vi "Main.vi"() -> ()   [LabVIEW 2020]
uses:
  TypeDefs/Enum_MainQueueElements.ctl
  TypeDefs/Refs_Common.ctl
  <vilib>/Stadlmann TEC/OXYGEN Datastream/VIs/Data Aquasation/TypeDefs/DataPoint_Double.ctl
  <vilib>/event_ctls.llb/eventvkey.ctl
  TypeDefs/TD_Case_SimpleFGVModes.ctl
  TypeDefs/Enum_CmdPromptActions.ctl
  <vilib>/Stadlmann TEC/OXYGEN Datastream/VIs/Setup/TypeDefs/States.ctl
  <vilib>/Stadlmann TEC/OXYGEN Datastream/VIs/Channel List Access/SubVIs/ChannelList_GetNames.vi
  <vilib>/Stadlmann TEC/OXYGEN Datastream/VIs/Setup/SubVIs/Start_Group.vi
  <vilib>/Stadlmann TEC/OXYGEN Datastream/VIs/Setup/SubVIs/Stop_Group.vi
  <vilib>/Stadlmann TEC/OXYGEN Datastream/VIs/Setup/SubVIs/Port_set.vi
  <vilib>/Stadlmann TEC/OXYGEN Datastream/VIs/Setup/SubVIs/Port_get.vi
  <vilib>/Stadlmann TEC/OXYGEN Datastream/VIs/Setup/SubVIs/Items_set.vi
  <vilib>/Stadlmann TEC/OXYGEN Datastream/VIs/Setup/SubVIs/Init_Group.vi
  <vilib>/Stadlmann TEC/OXYGEN Datastream/OXYGEN_Datastream.lvlib
  VIs/VI_ReadData.vi
panel:
  out "Bool_StatusLED":bool=TRUE
  in  "STR_HostAddress":string="127.0.0.1:10001"
  in  "Button_Disconnect":bool
  in  "Button_Connect":bool
  in  "Button_querryChs":bool
  in  "LBox_ChList":i32(listbox)
  in  "Datastream Port":u32=10003
  in  "Button_Set_Port":bool
  in  "Button_Reset":bool
  in  "Button_Init":bool
  in  "Button_Get_State":bool
  in  "Button_Get_Port":bool
  in  "Button_Start":bool
  in  "Button_Stop":bool
  in  "User Commands":string
  in  "STR_ChName1":string
  out "Num_ChValue1":dbl format="%04.3g"
  in  "STR_ChName2":string
  out "Num_ChValue2":dbl format="%1.3g"
  in  "STR_ChName3":string
  out "Num_ChValue3":dbl format="%1.3g"
  in  "STR_ChName4":string
  out "Num_ChValue4":dbl format="%.3g"
  in  "STR_ChName5":string
  out "Num_ChValue5":dbl format="%.3g"
  in  "STR_ChName6":string
  out "Num_ChValue6":dbl format="%.3g"
  out "Recorder":T1(graph)
  out "STR_CmdPrompt":string
  # "IP Address/Hostname and Port Number \n                Example:  xxx.xxx.xxx.xxx:yyyyy"
  # "Datastream Group 1"
  # "Channel 1"
  # "Channel 3"
  # "Channel 2"
  # "Channel 5"
  # "Channel 4"
  # "Channel 6"
  # "Channel 1"
  # "Channel 2"
  # "Channel 3"
  # "Channel 4"
  # "Channel 5"
  # "Channel 6"
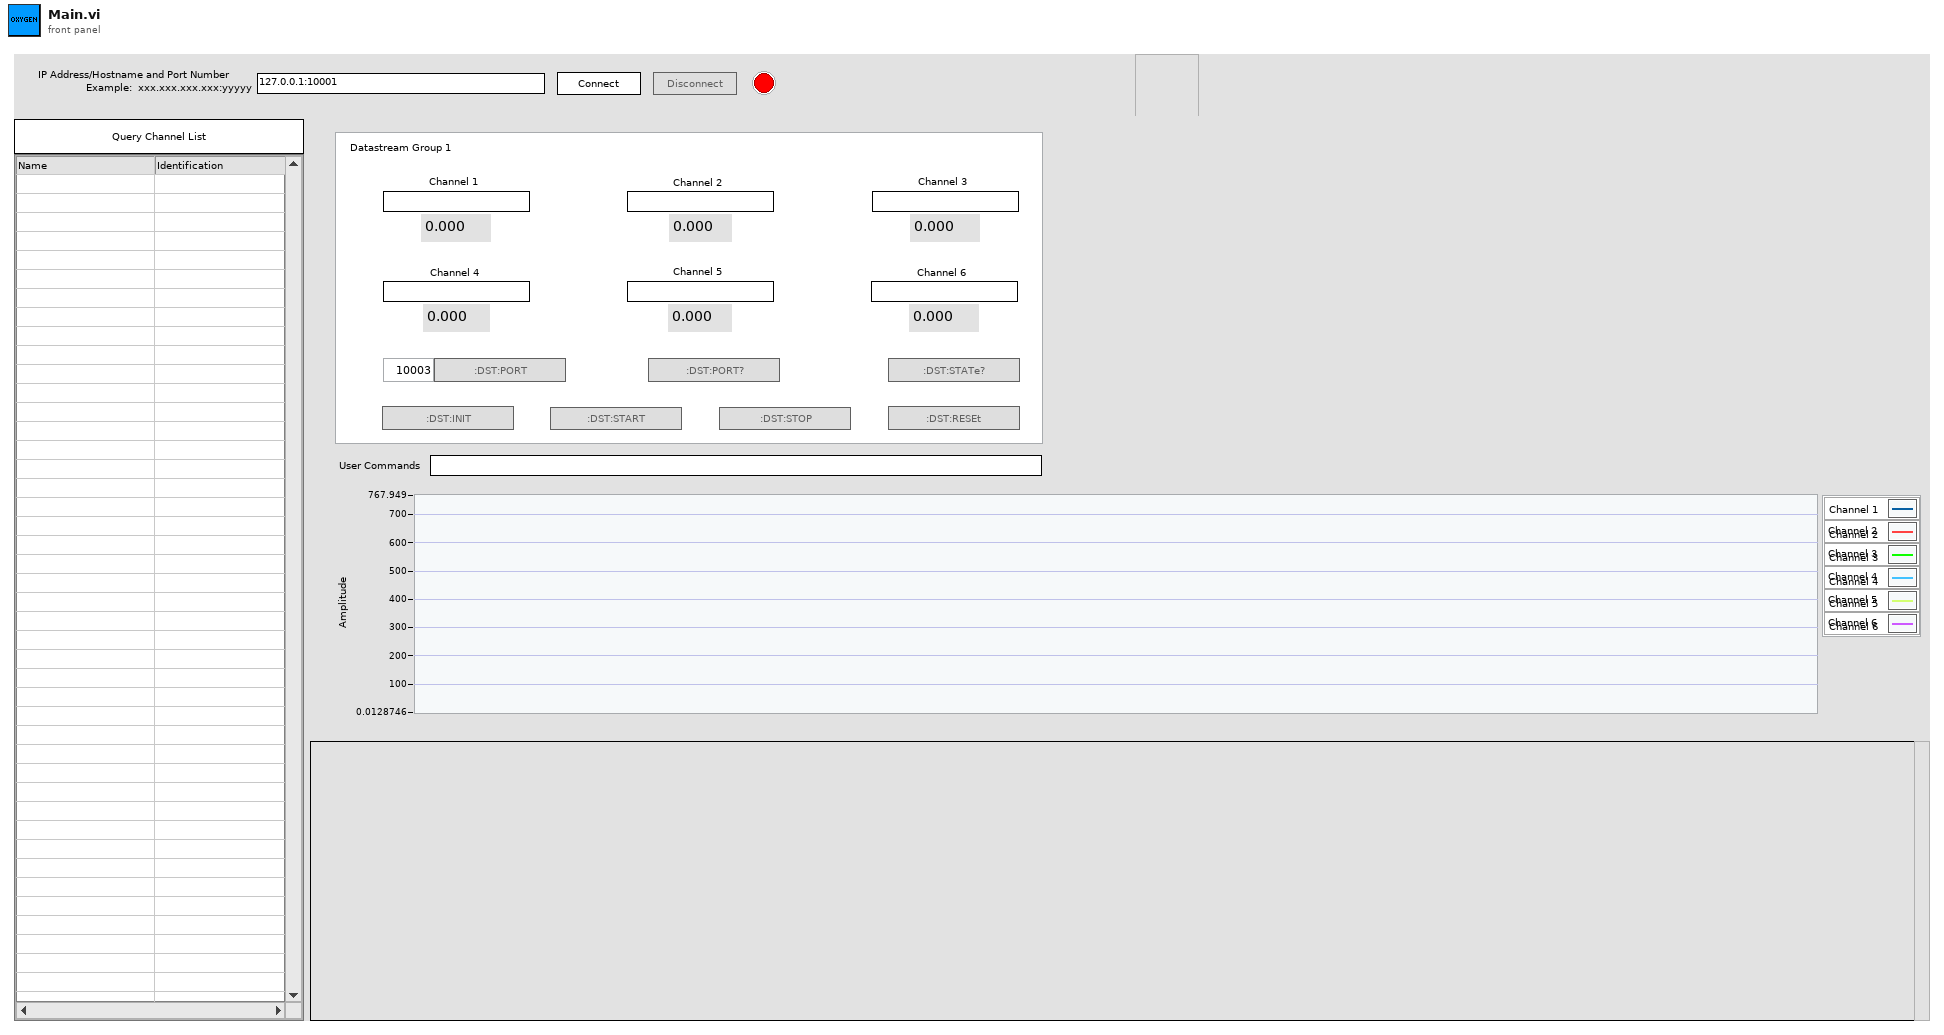
[diagram p1: front panel]
types:
  T1 = cluster{"DataPoints":cluster{"Value":dbl, "Time":dbl}[]}[]
  T2 = typedef "OXYGEN_Datastream.lvlib/DataPoint_Double.ctl" = cluster{"DataPoints":cluster{"Time":dbl, "Value":dbl}[]}
  T3 = typedef "Refs_Common.ctl" = cluster{"LBox_ChList":refnum<vi>, "OXY_SCPI Ref":refnum<visa-resource-name>, "STR_ChName1":refnum<vi>, "STR_ChName2":refnum<vi>, "STR_ChName3":refnum<vi>, "STR_ChName4":refnum<vi>, "STR_ChName5":refnum<vi>, "STR_ChName6":refnum<vi>, "Button_Stop":refnum<vi>, "Button_Start":refnum<vi>, "Button_Disconnect":refnum<vi>, "Button_Connect":refnum<vi>, "Bool_StatusLED":refnum<vi>, "DS Ref":refnum<visa-resource-name>, "Button_SetPort":refnum<vi>, "Button_GetPort":refnum<vi>, "Button_GetState":refnum<vi>, "Button_Reset":refnum<vi>, "Button_Init":refnum<vi>, "STR_UserCMD":refnum<vi>, "STR_CmdPromp":refnum<vi>, "Port":refnum<vi>, "Button_QuerryChs":refnum<vi>, "Graph":refnum<vi>, "STR_ConnAddress":refnum<vi>}
  T4 = typedef "Enum_MainQueueElements.ctl" = enum16{"Timeout", "Init", "Button_Reset_Pressed", "Button_QuerryChList_Pressed", "Button_UsrCmdSet_Pressed", "Button_StartTransfer_Pressed", "Button_StopTransfer_Pressed", "Button_Connect_Pressed", "Button_Disconnect_Pressed", "Button_SetPort_Presssed", "Button_GetPort_Pressed", "Button_GetState_Pressed", "Button_Init_Pressed", "NewDragAndDrop", "CloseApp"}
  T5 = typedef "Enum_CmdPromptActions.ctl" = enum16{"Init", "Add", "EditSettings", "Close"}
  T6 = cluster{"send_data":string, "received_data":string}
  T7 = typedef "OXYGEN_Datastream.lvlib/States.ctl" = enum16{"Invalid", "Config", "Initialized", "Running", "Error", "Unlicensed"}
  T8 = enum8{"Enabled", "Disabled", "Disabled and Grayed Out"}
  T9 = typedef "TD_Case_SimpleFGVModes.ctl" = enum16{"Set", "Get"}
  T10 = typedef "OXYGEN_Datastream.lvlib/Cluster_RawCommData.ctl" = cluster{"send_data":string, "received_data":string}
  T11 = typedef "eventvkey.ctl" = enum16{"ASCII", "Enter", "Return", "Shift", "Ctrl", "Alt", "Cmd", "Opt", "Caps", "NumLock", "Clear", "Break", "Up", "Down", "Left", "Right", "Insert", "Delete", "Home", "End", "PageUp", "PageDown", "Escape", "Help", "Pause", "ScrollLock", "F1", "F2", "F3", "F4", "F5", "F6", "F7", "F8", "F9", "F10", "F11", "F12", "F13", "F14", "F15", "F16", "F17", "F18", "F19", "F20", "F21", "F22", "F23", "F24", "Play", "VolumeUp", "VolumeDown", "Mute", "Two Byte Char"}
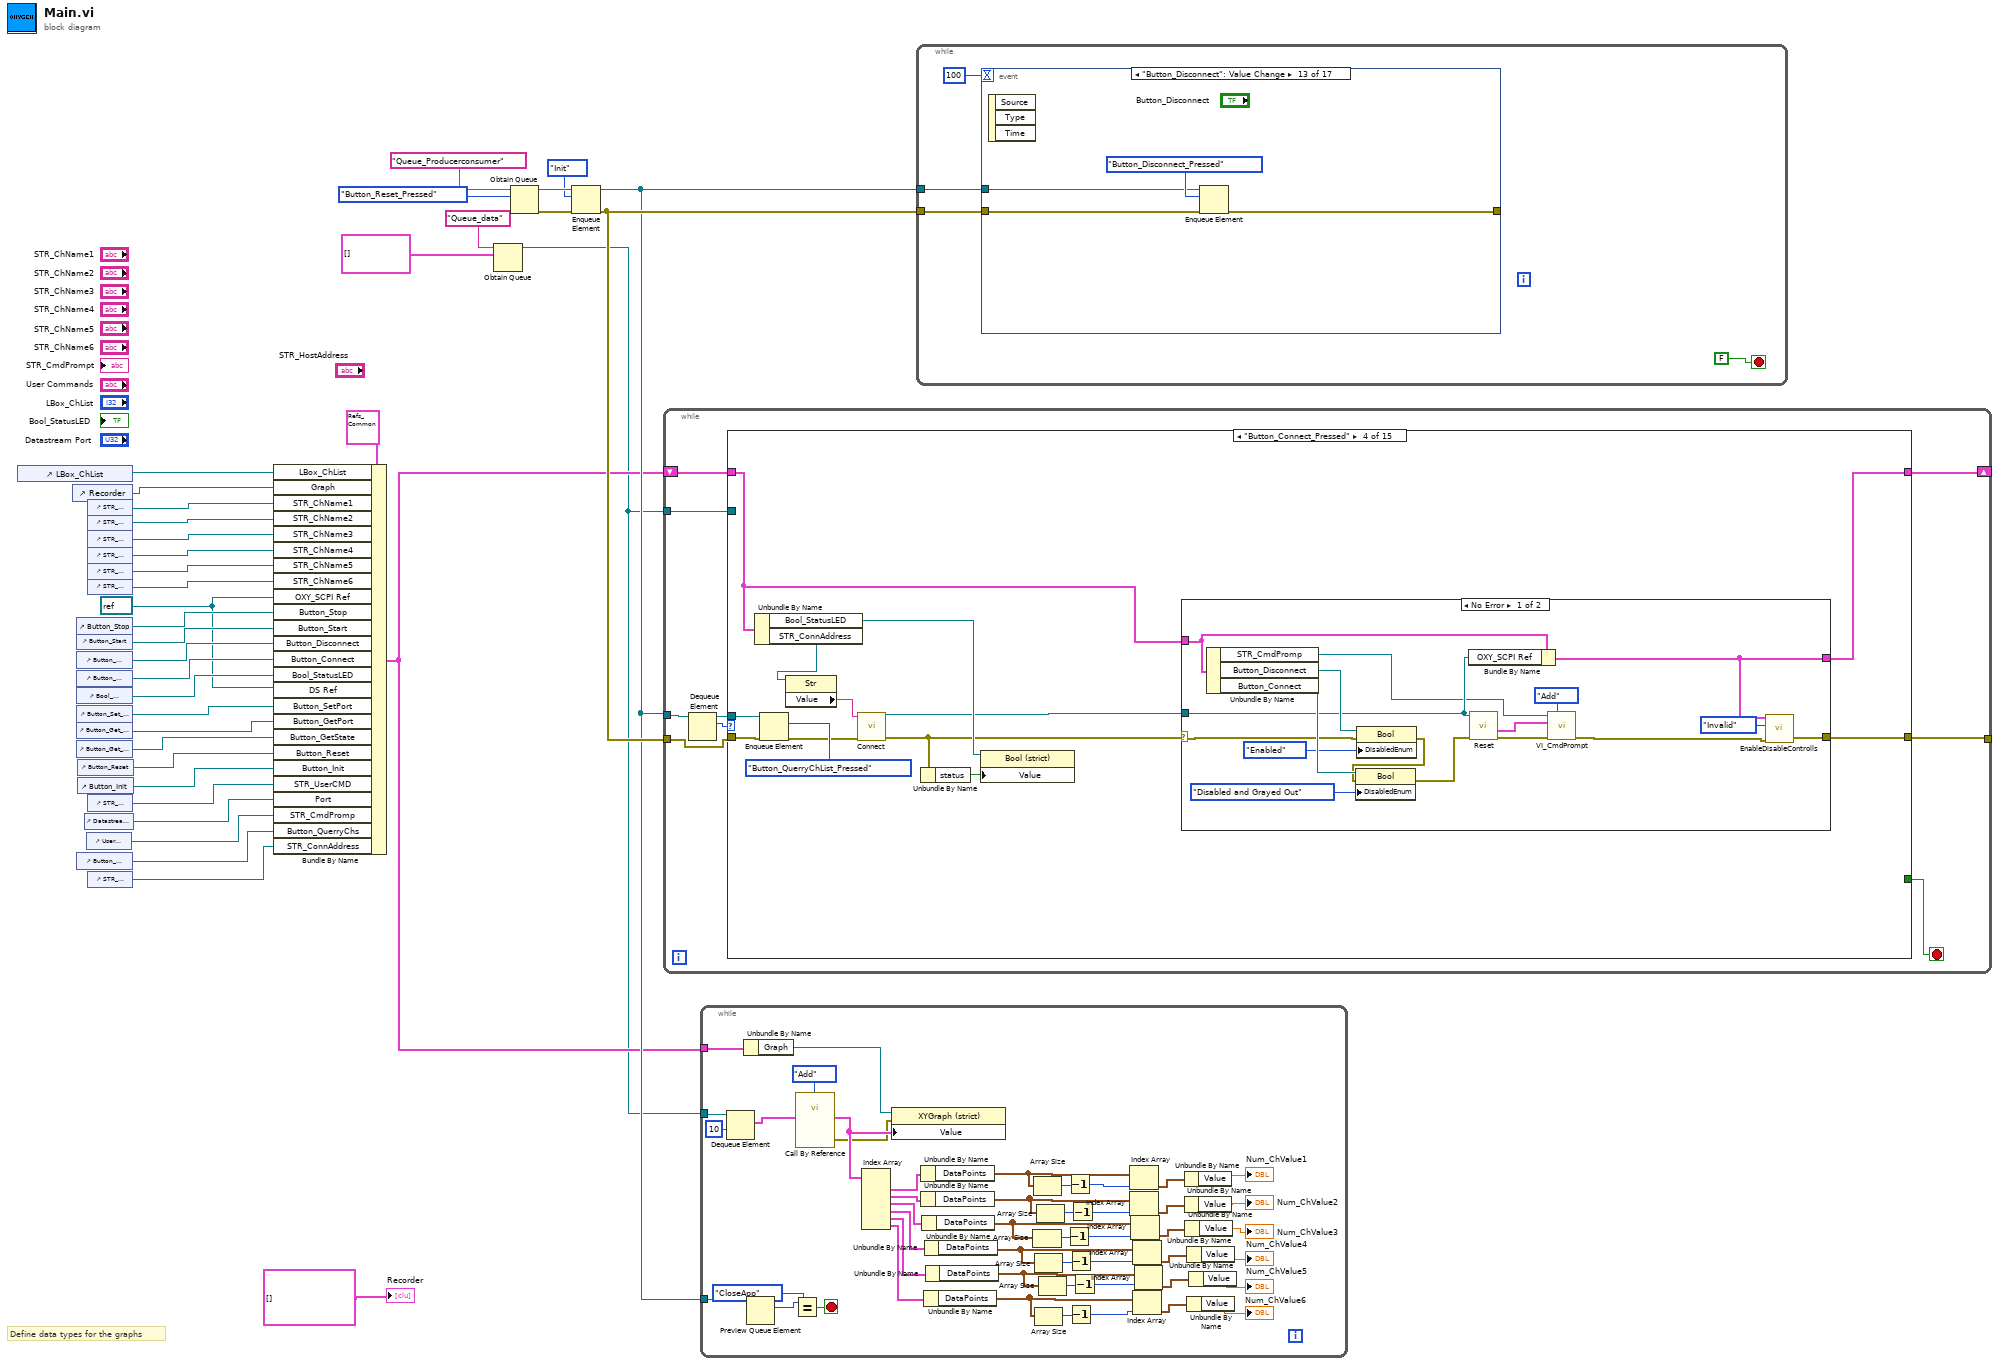
[diagram p0: block diagram]
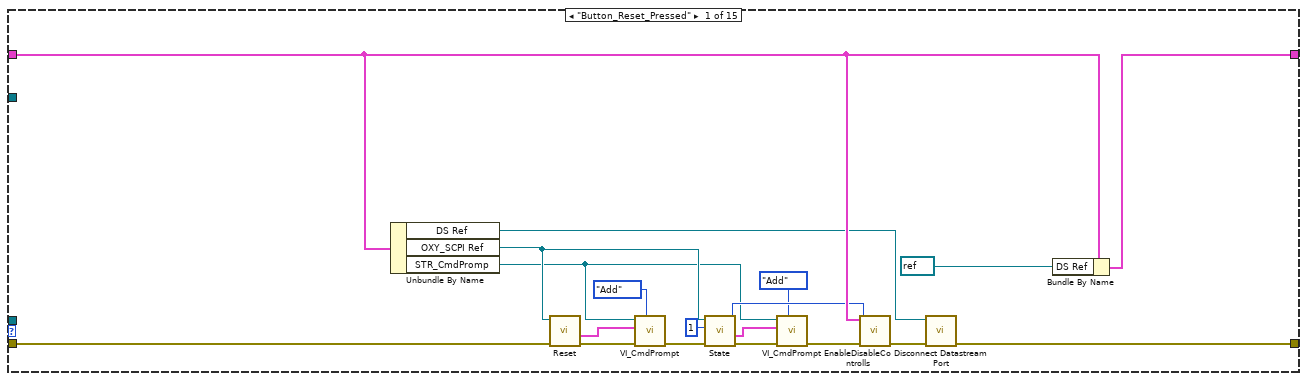
[diagram p2: hidden frame]
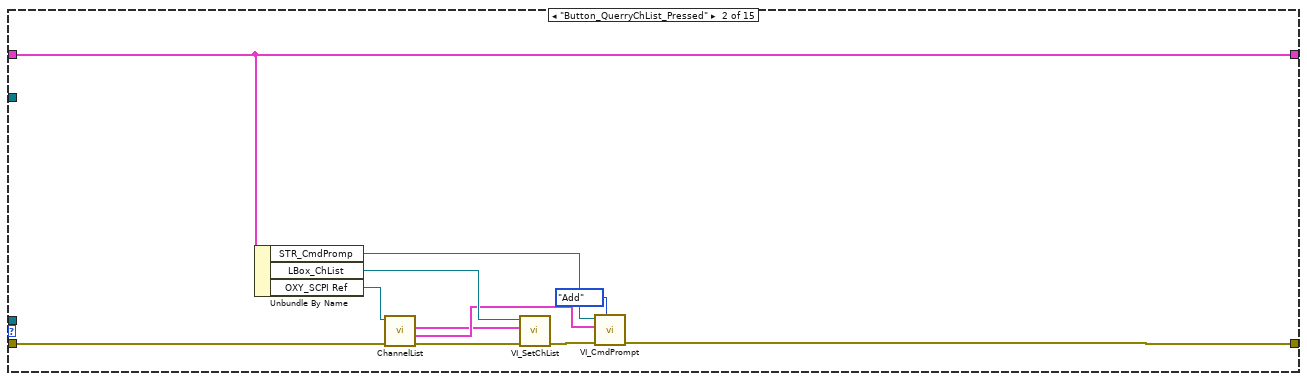
[diagram p3: hidden frame]
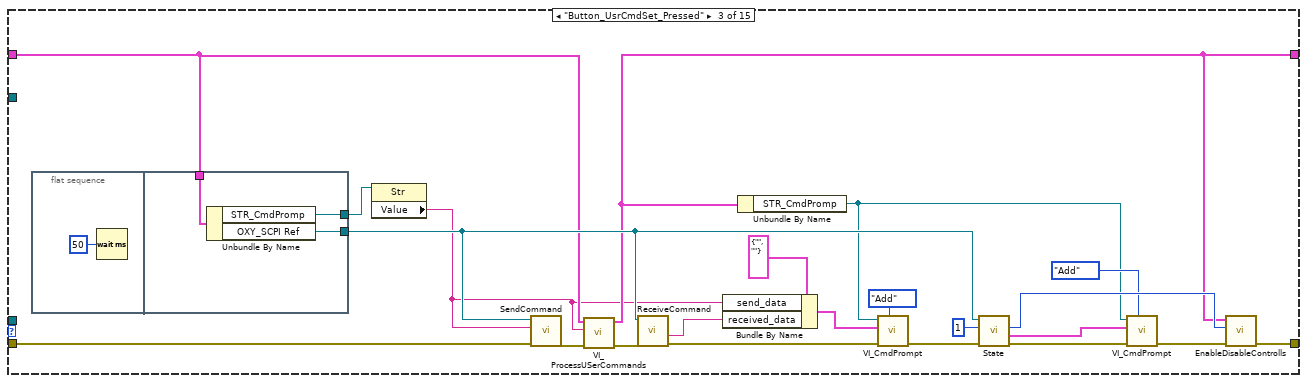
[diagram p4: hidden frame]
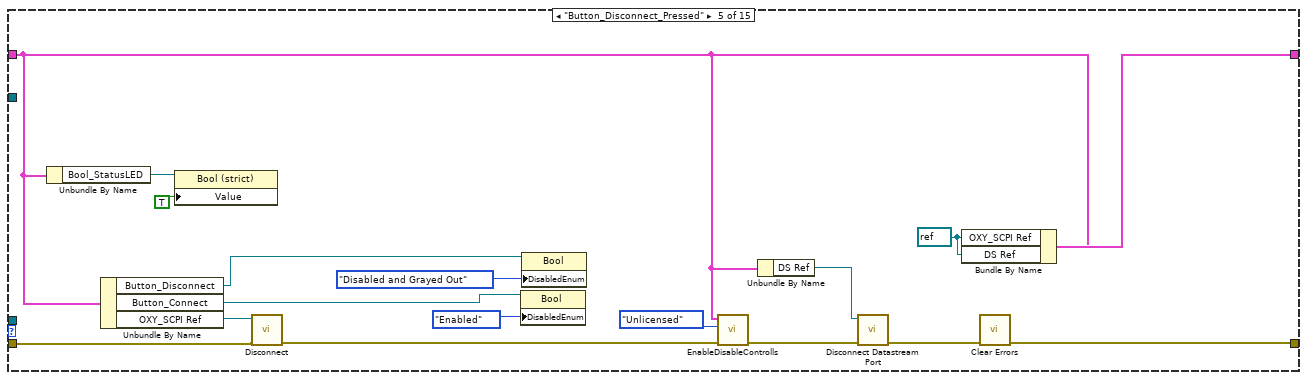
[diagram p6: hidden frame]
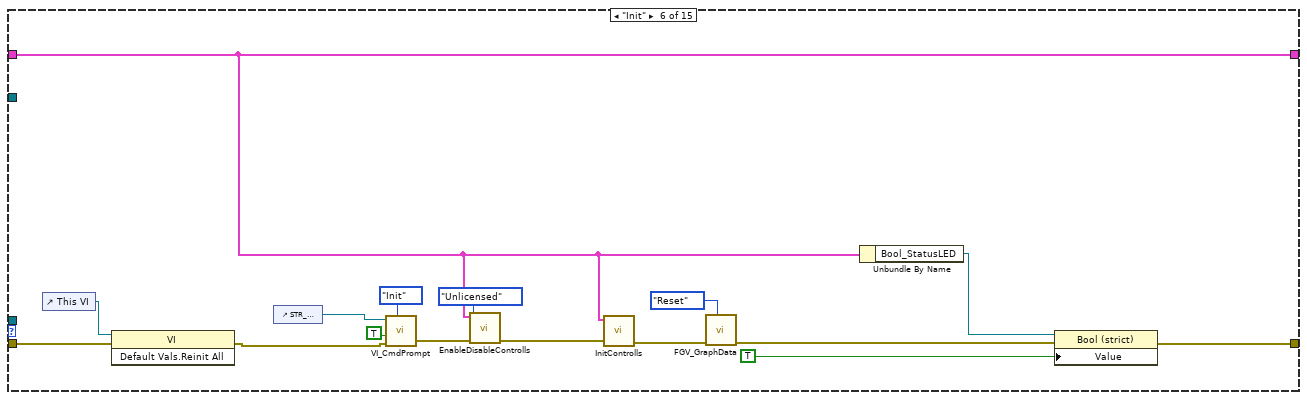
[diagram p7: hidden frame]
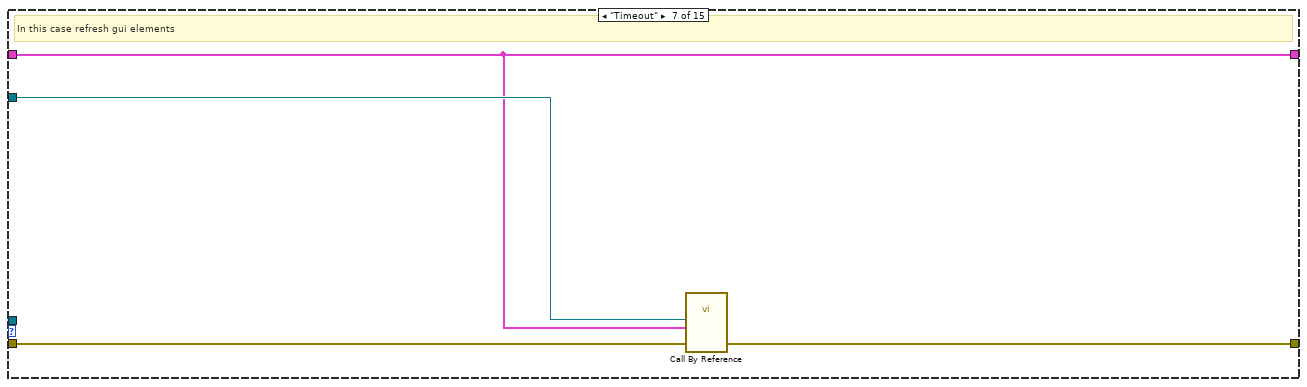
[diagram p8: hidden frame]
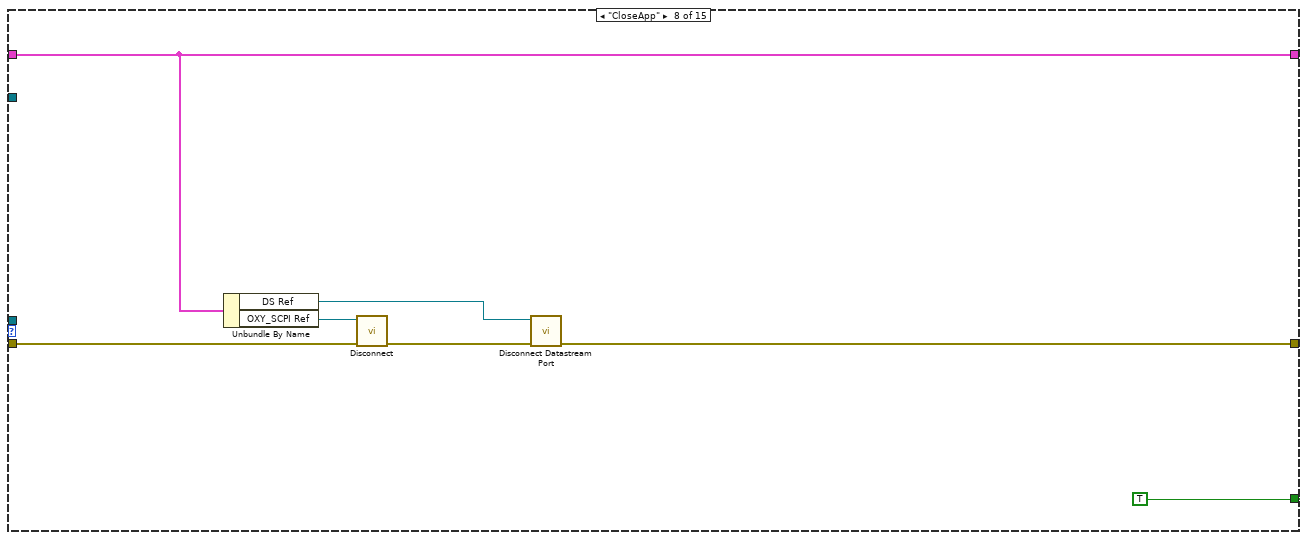
[diagram p9: hidden frame]
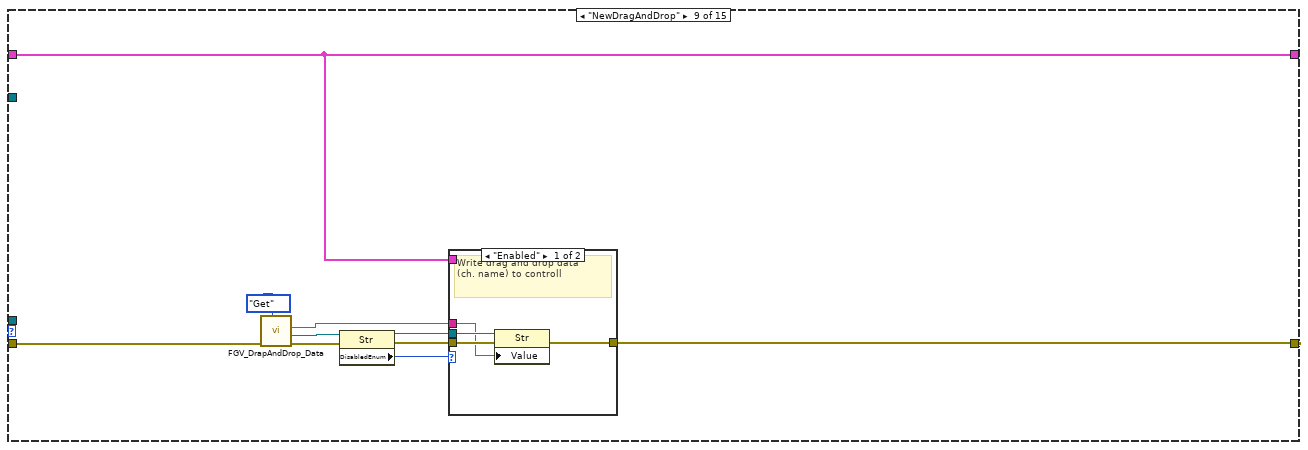
[diagram p10: hidden frame]
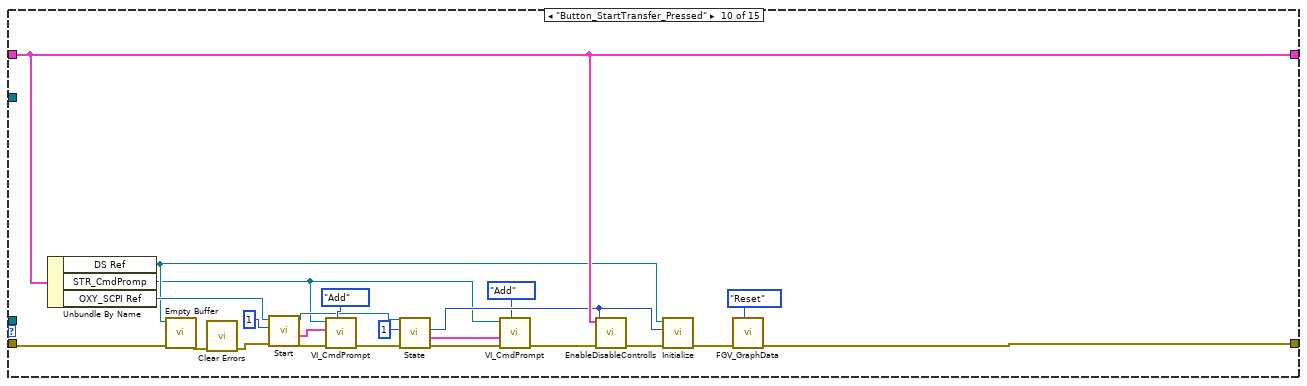
[diagram p12: hidden frame]
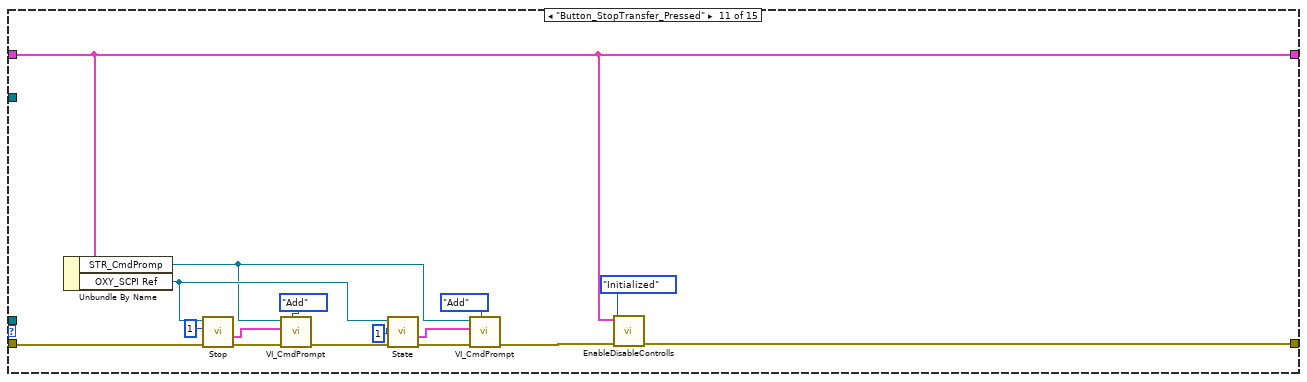
[diagram p13: hidden frame]
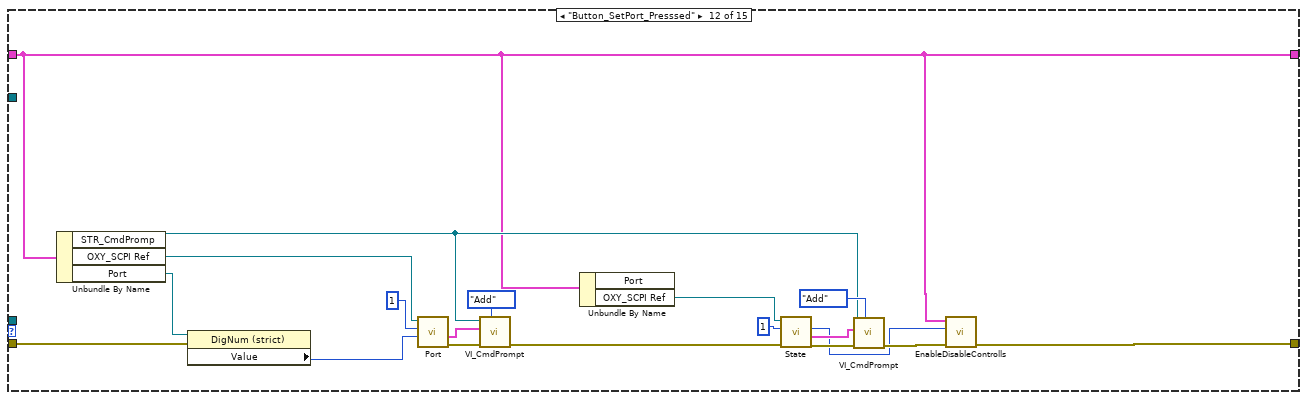
[diagram p14: hidden frame]
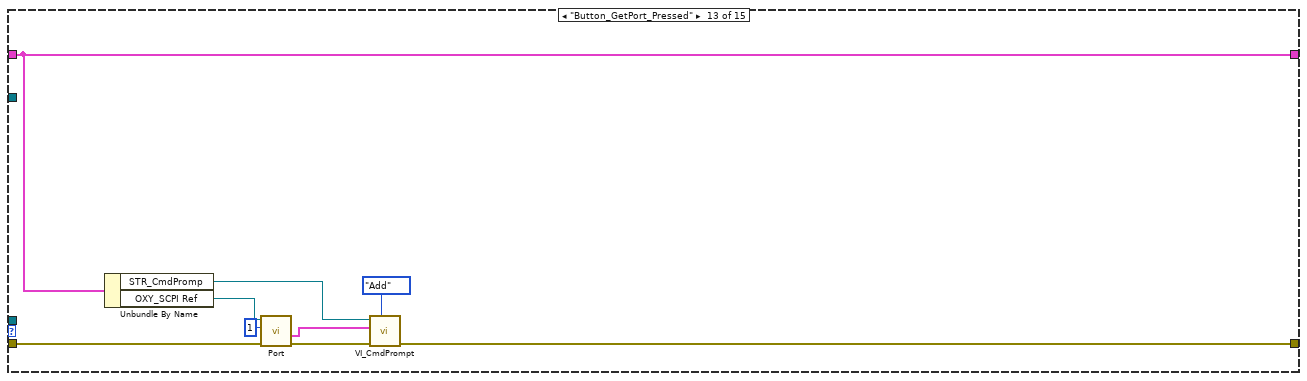
[diagram p15: hidden frame]
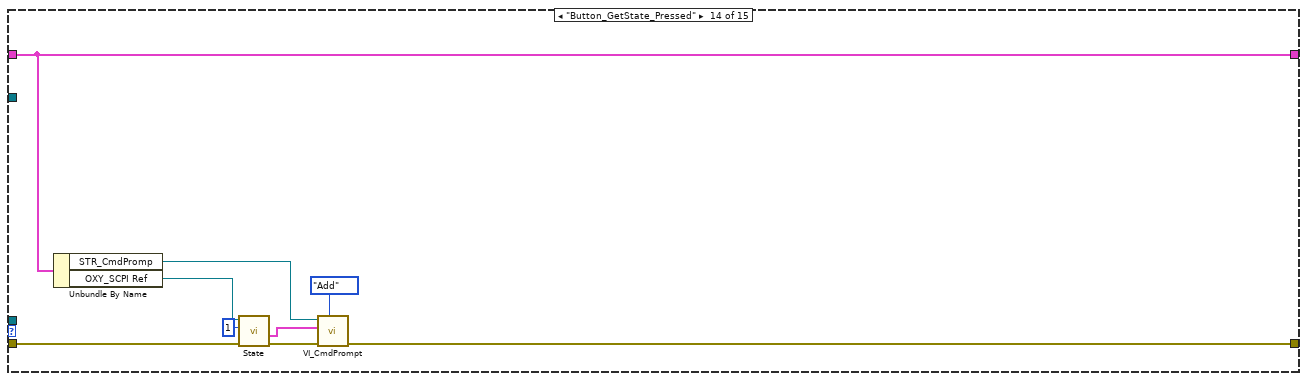
[diagram p16: hidden frame]
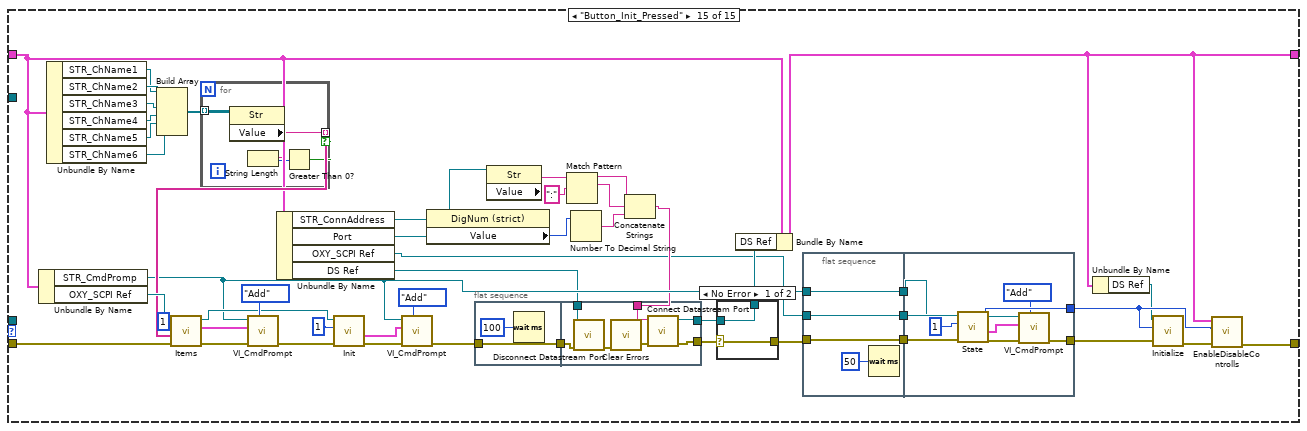
[diagram p17: hidden frame]
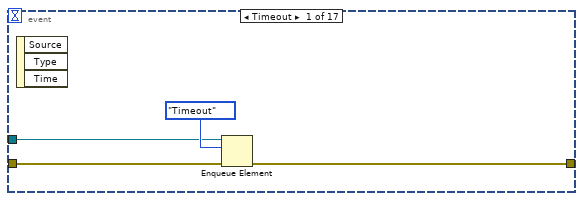
[diagram p19: hidden frame]
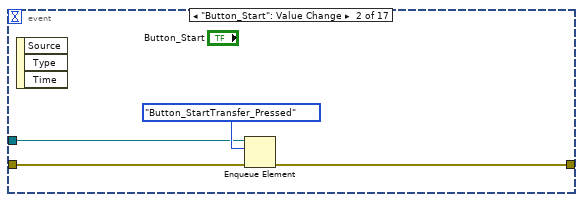
[diagram p20: hidden frame]
diagram:
  w12 = refnum<visa-resource-name> refnum ("OXY_SCPI Ref")
  # "Define data types for the graphs"
  n1 = control-ref of="LBox_ChList"() -> (w25:refnum<vi>)
  n2 = control-ref of="Recorder"() -> (w23:refnum<vi>)
  n3 = control-ref of="Button_Stop"() -> (w22:refnum<vi>)
  n4 = control-ref of="Button_Start"() -> (w21:refnum<vi>)
  n5 = control-ref of="Button_Disconnect"() -> (w20:refnum<vi>)
  n6 = control-ref of="Button_Connect"() -> (w19:refnum<vi>)
  n7 = control-ref of="Bool_StatusLED"() -> (w18:refnum<vi>)
  n8 = control-ref of="Button_Set_Port"() -> (w17:refnum<vi>)
  n9 = control-ref of="Button_Get_Port"() -> (w16:refnum<vi>)
  n10 = control-ref of="Button_Get_State"() -> (w13:refnum<vi>)
  n11 = control-ref of="Button_querryChs"() -> (w8:refnum<vi>)
  n12 = control-ref of="Button_Reset"() -> (w15:refnum<vi>)
  n13 = control-ref of="Button_Init"() -> (w14:refnum<vi>)
  n14 = control-ref of="Datastream Port"() -> (w9:refnum<vi>)
  n15 = control-ref of="User Commands"() -> (w10:refnum<vi>)
  n16 = control-ref of="STR_ChName1"() -> (w26:refnum<vi>)
  n17 = control-ref of="STR_ChName2"() -> (w27:refnum<vi>)
  n18 = control-ref of="STR_ChName3"() -> (w28:refnum<vi>)
  n19 = control-ref of="STR_ChName4"() -> (w29:refnum<vi>)
  n20 = control-ref of="STR_ChName5"() -> (w30:refnum<vi>)
  n21 = control-ref of="STR_ChName6"() -> (w31:refnum<vi>)
  n22 = control-ref of="STR_CmdPrompt"() -> (w11:refnum<vi>)
  n23 = control-ref of="STR_HostAddress"() -> (w6:refnum<vi>)
  n24 = Bundle By Name(cluster=T3 {"LBox_ChList"=refnum, "OXY_SCPI Ref"="", "STR_ChName1"=refnum, "STR_ChName2"=refnum, "STR_ChName3"=refnum, "STR_ChName4"=refnum, "STR_ChName5"=refnum, "STR_ChName6"=refnum, "Button_Stop"=refnum, "Button_Start"=refnum, "Button_Disconnect"=refnum, "Button_Connect"=refnum, "Bool_StatusLED"=refnum, "DS Ref"="", "Button_SetPort"=refnum, "Button_GetPort"=refnum, "Button_GetState"=refnum, "Button_Reset"=refnum, "Button_Init"=refnum, "STR_UserCMD"=refnum, "STR_CmdPromp"=refnum, "Port"=refnum, "Button_QuerryChs"=refnum, "Graph"=refnum, "STR_ConnAddress"=refnum} ("Common Refs"), "LBox_ChList"=w25, "Graph"=w23, "STR_ChName1"=w26, "STR_ChName2"=w27, "STR_ChName3"=w28, "STR_ChName4"=w29, "STR_ChName5"=w30, "STR_ChName6"=w31, "OXY_SCPI Ref"=w12, "Button_Stop"=w22, "Button_Start"=w21, "Button_Disconnect"=w20, "Button_Connect"=w19, "Bool_StatusLED"=w18, "DS Ref"=w12, "Button_SetPort"=w17, "Button_GetPort"=w16, "Button_GetState"=w13, "Button_Reset"=w15, "Button_Init"=w14, "STR_UserCMD"=w11, "Port"=w9, "STR_CmdPromp"=w10, "Button_QuerryChs"=w8, "STR_ConnAddress"=w6) -> (w3:T3)
  n25 = Obtain Queue(name (unnamed)="Queue_data", element data type=T2[] [] ("Data")) -> (queue out=w2:refnum<queue>)  [unwired: 3 in, 2 out]
  n26 = Obtain Queue(name (unnamed)="Queue_Producerconsumer", element data type=Enum_MainQueueElements."Button_Reset_Pressed") -> (queue out=w35:refnum<queue>, error out=w33:errorcluster)  [unwired: 3 in, 1 out]
  n27 = Enqueue Element(queue=w35, element=Enum_MainQueueElements."Init", error in (no error)=w33) -> (queue out=w5:refnum<queue>, error out=w34:errorcluster)  [unwired: 1 in, 1 out]
  n28 = while {
    tunnel: w5 -> [w41]
    shift-right: [w43] -> _
    shift-left: w3 -> [w44]
    tunnel: w2 -> [w42]
    tunnel: w34 -> [w39]
    tunnel: [w40] -> _
    stop <- w45 stop-if-true
    n29 = Dequeue Element(queue=w41) -> (queue out=w38:refnum<queue>, element=w46:T4)  [unwired: 2 in, 2 out]
    n30 = case shown="\"Button_Connect_Pressed\"" w46 {
      tunnel: w39 -> [w62 w68 w94 w104 w144 w161 w168 w176 w181 w205 w228 w245 w259 w269 w302]
      tunnel: [w47 w73 w88 w110 w135 w160 w171 w174 w180 w206 w225 w244 w252 w266 w298] -> w40
      tunnel: w44 -> [w59 w75 w87 w109 w141 w158 w169 w178 w179 w207 w224 w234 w257 w265 w274]
      tunnel: [_ _ _ _ _ _ _ TRUE _ _ _ _ _ _ _] -> w45
      tunnel: [w60 w75 w84 w111 w147 w158 w169 w178 w179 w207 w224 w234 w257 w265 w276] -> w43
      tunnel: w42 -> [_ _ _ _ _ _ w170 _ _ _ _ _ _ _ _]
      tunnel: w38 -> [_ _ _ w103 _ _ _ _ _ _ _ _ _ _ _]
      frame "Button_Reset_Pressed" {
        n31 = Unbundle By Name(w59) -> ("DS Ref"=w48:refnum<visa-resource-name>, "OXY_SCPI Ref"=w58:refnum<visa-resource-name>, "STR_CmdPromp"=w53:refnum<vi>)
        n32 = call <vilib>:"Reset.vi"("error in (no error)"=w62, "OXY_SCPI Reseource In"=w58) -> ("error out"=w64:errorcluster, "communication_data"=w63:T10)  [unwired: 7 in, 1 out]
        n33 = call "VI_CmdPrompt.vi"("Mode"=Enum_CmdPromptActions."Add", "error in (no error)"=w64, "communication_data"=w63, "STR_CmdPrompt_Ref"=w53) -> ("error out"=w57:errorcluster)  [unwired: 7 in]
        n34 = call <vilib>:"State.vi"("error in (no error)"=w57, "Group"=1, "OXY_SCPI Reseource In"=w58) -> ("error out"=w51:errorcluster, "communication_data"=w52:T10, "State"=w56:T7)  [unwired: 5 in, 1 out]
        n35 = call "VI_CmdPrompt.vi"("Mode"=Enum_CmdPromptActions."Add", "error in (no error)"=w51, "communication_data"=w52, "STR_CmdPrompt_Ref"=w53) -> ("error out"=w50:errorcluster)  [unwired: 7 in]
        n36 = call "EnableDisableControlls.vi"("error in (no error)"=w50, "State"=w56, "Common Refs"=w59) -> ("error out"=w49:errorcluster)  [unwired: 8 in]
        n37 = call <vilib>:"Disconnect Datastream Port.vi"("error in (no error)"=w49, "OXY_SCPI Reseource Out"=w48) -> ("error out"=w47:errorcluster)  [unwired: 9 in]
        n38 = Bundle By Name(cluster=w59, "DS Ref"=refnum<visa-resource-name> refnum) -> (w60:T3)
      }
      frame "Button_QuerryChList_Pressed" {
        n39 = Unbundle By Name(w75) -> ("STR_CmdPromp"=w66:refnum<vi>, "LBox_ChList"=w72:refnum<vi>, "OXY_SCPI Ref"=w69:refnum<visa-resource-name>)
        n40 = call-poly <vilib>:"ChannelList.vi"("error in (no error)"=w68, "OXY_SCPI Reseource In"=w69) -> ("error out"=w67:errorcluster, "communication_data"=w71:T10, "Channels"=w70:cluster{"ID":string, "Name":string}[])  [unwired: 6 in, 1 out]
        n41 = call "VI_SetChList.vi"("error in (no error)"=w67, "Channel List"=w70, "ChList_Ref In"=w72) -> ("error out"=w74:errorcluster)  [unwired: 7 in, 1 out]
        n42 = call "VI_CmdPrompt.vi"("Mode"=Enum_CmdPromptActions."Add", "error in (no error)"=w74, "communication_data"=w71, "STR_CmdPrompt_Ref"=w66) -> ("error out"=w73:errorcluster)  [unwired: 7 in]
      }
      frame "Button_UsrCmdSet_Pressed" {
        n43 = flat-sequence {
          tunnel: w87 -> [w102]
          tunnel: [w101] -> w91
          tunnel: [w100] -> w83
          frame #0 {
            n44 = Wait (ms)(milliseconds to wait=u32 50) -> ()  [unwired: 1 out]
          }
          frame #1 {
            n45 = Unbundle By Name(w102) -> ("STR_CmdPromp"=w100:refnum<vi>, "OXY_SCPI Ref"=w101:refnum<visa-resource-name>)
          }
        }
        n46 = property class="Str"(reference=w83) -> ("Value"=w82:string)  [unwired: 1 in, 2 out]
        n47 = call <vilib>:"SendCommand.vi"("error in (no error)"=w94, "String to Send"=w82, "OXY_SCPI Reseource In"=w91) -> ("error out"=w86:errorcluster)  [unwired: 7 in, 1 out]
        n48 = call "VI_ProcessUSerCommands.vi"("error in (no error)"=w86, "send command"=w82, "Common Refs"=w87) -> ("error out"=w85:errorcluster, "Common Refs 2"=w84:T3)  [unwired: 7 in]
        n49 = call <vilib>:"ReceiveCommand.vi"("error in (no error)"=w85, "OXY_SCPI Reseource In"=w91) -> ("error out"=w95:errorcluster, "received Data with Header"=w93:string)  [unwired: 6 in, 2 out]
        n50 = Bundle By Name(cluster=T6 {"send_data"="", "received_data"=""} ("communication_data"), "send_data"=w82, "received_data"=w93) -> (w96:T6)
        n51 = Unbundle By Name(w84) -> ("STR_CmdPromp"=w77:refnum<vi>)
        n52 = call "VI_CmdPrompt.vi"("Mode"=Enum_CmdPromptActions."Add", "error in (no error)"=w95, "communication_data"=w96, "STR_CmdPrompt_Ref"=w77) -> ("error out"=w90:errorcluster)  [unwired: 7 in]
        n53 = call <vilib>:"State.vi"("error in (no error)"=w90, "Group"=1, "OXY_SCPI Reseource In"=w91) -> ("error out"=w78:errorcluster, "communication_data"=w80:T10, "State"=w89:T7)  [unwired: 5 in, 1 out]
        n54 = call "VI_CmdPrompt.vi"("Mode"=Enum_CmdPromptActions."Add", "error in (no error)"=w78, "communication_data"=w80, "STR_CmdPrompt_Ref"=w77) -> ("error out"=w79:errorcluster)  [unwired: 7 in]
        n55 = call "EnableDisableControlls.vi"("error in (no error)"=w79, "State"=w89, "Common Refs"=w84) -> ("error out"=w88:errorcluster)  [unwired: 8 in]
      }
      frame "Button_Connect_Pressed" {
        n56 = Unbundle By Name(w109) -> ("Bool_StatusLED"=w115:refnum<vi>, "STR_ConnAddress"=w108:refnum<vi>)
        n57 = Enqueue Element(queue=w103, element=Enum_MainQueueElements."Button_QuerryChList_Pressed", error in (no error)=w104) -> (error out=w105:errorcluster)  [unwired: 1 in, 2 out]
        n58 = property class="Str"(reference=w108) -> ("Value"=w107:string)  [unwired: 1 in, 2 out]
        n59 = call <vilib>:"Connect.vi"("error in (no error)"=w105, "OXY_SCPI Resource In"=w107) -> ("error out"=w113:errorcluster, "OXY_SCPI Resource Out"=w112:refnum<visa-resource-name>)  [unwired: 8 in]
        n60 = Unbundle By Name(w113) -> ("status"=w114:bool)
        n61 = property class="Bool (strict)"(reference=w115, "Value"=w114) -> ()  [unwired: 1 in, 2 out]
        n62 = case shown="No Error" w113 {
          selector: w113 -> [w128 w134]
          tunnel: [w122 w134] -> w110
          tunnel: w109 -> [w126 w133]
          tunnel: [w121 w133] -> w111
          tunnel: w112 -> [w120 _]
          frame No Error {
            n63 = Unbundle By Name(w126) -> ("STR_CmdPromp"=w118:refnum<vi>, "Button_Disconnect"=w132:refnum<vi>, "Button_Connect"=w131:refnum<vi>)
            n64 = property class="Bool"(reference=w132, error in=w128, "DisabledEnum"=T8."Enabled" ("Disabled")) -> (error out=w127:errorcluster)  [unwired: 1 out]
            n65 = property class="Bool"(reference=w131, error in=w127, "DisabledEnum"=T8."Disabled and Grayed Out" ("Disabled")) -> (error out=w119:errorcluster)  [unwired: 1 out]
            n66 = Bundle By Name(cluster=w126, "OXY_SCPI Ref"=w120) -> (w121:T3)
            n67 = call <vilib>:"Reset.vi"("error in (no error)"=w119, "OXY_SCPI Reseource In"=w120) -> ("error out"=w124:errorcluster, "communication_data"=w123:T10)  [unwired: 7 in, 1 out]
            n68 = call "VI_CmdPrompt.vi"("Mode"=Enum_CmdPromptActions."Add", "error in (no error)"=w124, "communication_data"=w123, "STR_CmdPrompt_Ref"=w118) -> ("error out"=w117:errorcluster)  [unwired: 7 in]
            n69 = call "EnableDisableControlls.vi"("error in (no error)"=w117, "State"=States."Invalid", "Common Refs"=w121) -> ("error out"=w122:errorcluster)  [unwired: 8 in]
          }
          frame Error {
          }
        }
      }
      frame "Button_Disconnect_Pressed" {
        w137 = refnum<visa-resource-name> refnum ("OXY_SCPI Ref")
        n70 = Unbundle By Name(w141) -> ("Bool_StatusLED"=w146:refnum<vi>)
        n71 = Unbundle By Name(w141) -> ("Button_Disconnect"=w149:refnum<vi>, "Button_Connect"=w148:refnum<vi>, "OXY_SCPI Ref"=w143:refnum<visa-resource-name>)
        n72 = property class="Bool (strict)"(reference=w146, "Value"=TRUE) -> ()  [unwired: 1 in, 2 out]
        n73 = call <vilib>:"Disconnect.vi"("error in (no error)"=w144, "OXY_SCPI Reseource Out"=w143) -> ("error out"=w142:errorcluster)  [unwired: 9 in]
        n74 = property class="Bool"(reference=w148, "DisabledEnum"=T8."Enabled" ("Disabled")) -> ()  [unwired: 1 in, 2 out]
        n75 = property class="Bool"(reference=w149, "DisabledEnum"=T8."Disabled and Grayed Out" ("Disabled")) -> ()  [unwired: 1 in, 2 out]
        n76 = call "EnableDisableControlls.vi"("error in (no error)"=w142, "State"=States."Unlicensed", "Common Refs"=w141) -> ("error out"=w138:errorcluster)  [unwired: 8 in]
        n77 = Unbundle By Name(w141) -> ("DS Ref"=w139:refnum<visa-resource-name>)
        n78 = call <vilib>:"Disconnect Datastream Port.vi"("error in (no error)"=w138, "OXY_SCPI Reseource Out"=w139) -> ("error out"=w136:errorcluster)  [unwired: 9 in]
        n79 = Bundle By Name(cluster=w141, "OXY_SCPI Ref"=w137, "DS Ref"=w137) -> (w147:T3)
        n80 = call <vilib>:"Clear Errors.vi"("error in (no error)"=w136) -> ("error out"=w135:errorcluster)  [unwired: 5 in, 1 out]
      }
      frame "Init" {
        n81 = control-ref of="This VI"() -> (w162:refnum<vi>)
        n82 = invoke class="VI" method="Default Vals.Reinit All"(reference=w162, error in=w161) -> (error out=w159:errorcluster)  [unwired: 1 in, 2 out]
        n83 = control-ref of="STR_CmdPrompt"() -> (w166:refnum<vi>)
        n84 = call "VI_CmdPrompt.vi"("Mode"=Enum_CmdPromptActions."Init", "error in (no error)"=w159, "Activate?"=TRUE, "STR_CmdPrompt_Ref"=w166) -> ("error out"=w157:errorcluster)  [unwired: 7 in]
        n85 = call "EnableDisableControlls.vi"("error in (no error)"=w157, "State"=States."Unlicensed", "Common Refs"=w158) -> ("error out"=w156:errorcluster)  [unwired: 8 in]
        n86 = call "InitControlls.vi"("error in (no error)"=w156, "Common Refs"=w158) -> ("error out"=w153:errorcluster)  [unwired: 9 in]
        n87 = call "FGV_GraphData.vi"("Mode"=enum16{"Reset", "Add", "Get"}."Reset", "error in (no error)"=w153) -> ("error out"=w154:errorcluster)  [unwired: 8 in, 1 out]
        n88 = Unbundle By Name(w158) -> ("Bool_StatusLED"=w164:refnum<vi>)
        n89 = property class="Bool (strict)"(reference=w164, error in=w154, "Value"=TRUE) -> (error out=w160:errorcluster)  [unwired: 1 out]
      }
      frame "Timeout" {
        # "In this case refresh gui elements"
        n90 = call-by-ref "?"("error in (no error)"=w168, "Common Refs"=w169, "queue"=w170) -> ("error out"=w171:errorcluster)  [unwired: 10 in, 2 out]
      }
      frame "CloseApp" {
        n91 = Unbundle By Name(w178) -> ("DS Ref"=w172:refnum<visa-resource-name>, "OXY_SCPI Ref"=w175:refnum<visa-resource-name>)
        n92 = call <vilib>:"Disconnect.vi"("error in (no error)"=w176, "OXY_SCPI Reseource Out"=w175) -> ("error out"=w173:errorcluster)  [unwired: 9 in]
        n93 = call <vilib>:"Disconnect Datastream Port.vi"("error in (no error)"=w173, "OXY_SCPI Reseource Out"=w172) -> ("error out"=w174:errorcluster)  [unwired: 9 in]
      }
      frame "NewDragAndDrop" {
        n94 = call "FGV_DrapAndDrop_Data.vi"("Modes"=TD_Case_SimpleFGVModes."Get", "error in (no error)"=w181) -> ("error out"=w187:errorcluster, "Target String Element Ref Out"=w186:refnum<vi>, "Channel Name Out"=w182:string)  [unwired: 7 in]
        n95 = property class="Str"(reference=w186, error in=w187) -> (reference out=w185:refnum<vi>, error out=w184:errorcluster, "DisabledEnum"=w183:T8)
        n96 = case shown="\"Enabled\"" w183 {
          tunnel: w185 -> [w192 _]
          tunnel: w184 -> [w191 w193]
          tunnel: w182 -> [w190 _]
          tunnel: [w189 w193] -> w180
          tunnel: w179 -> [_ _]
          frame "Enabled" {
            # "Write drag and drop data\n(ch. name) to controll"
            n97 = property class="Str"(reference=w192, error in=w191, "Value"=w190) -> (error out=w189:errorcluster)  [unwired: 1 out]
          }
          frame "Disabled", Default {
            # "Do not place drag and drop data (ch name) if controll is diabled"
          }
        }
      }
      frame "Button_StartTransfer_Pressed" {
        n98 = Unbundle By Name(w207) -> ("DS Ref"=w203:refnum<visa-resource-name>, "STR_CmdPromp"=w199:refnum<vi>, "OXY_SCPI Ref"=w215:refnum<visa-resource-name>)
        n99 = call <vilib>:"Empty Buffer.vi"("error in (no error)"=w205, "OXY_SCPI Reseource In"=w203) -> ("error out"=w194:errorcluster)  [unwired: 8 in, 1 out]
        n100 = call <vilib>:"Clear Errors.vi"("error in (no error)"=w194) -> ("error out"=w195:errorcluster)  [unwired: 5 in, 1 out]
        n101 = call-poly <vilib>:"Start.vi"("error in (no error)"=w195, "Stream Group"=1, "OXY_SCPI Reseource In"=w215) -> ("error out"=w213:errorcluster, "communication_data"=w212:T10, "OXY_SCPI Reseource Out"=w209:refnum<visa-resource-name>)  [unwired: 6 in]
        n102 = call "VI_CmdPrompt.vi"("Mode"=Enum_CmdPromptActions."Add", "error in (no error)"=w213, "communication_data"=w212, "STR_CmdPrompt_Ref"=w199) -> ("error out"=w210:errorcluster)  [unwired: 7 in]
        n103 = call <vilib>:"State.vi"("error in (no error)"=w210, "Group"=1, "OXY_SCPI Reseource In"=w209) -> ("error out"=w197:errorcluster, "communication_data"=w198:T10, "State"=w201:T7)  [unwired: 5 in, 1 out]
        n104 = call "VI_CmdPrompt.vi"("Mode"=Enum_CmdPromptActions."Add", "error in (no error)"=w197, "communication_data"=w198, "STR_CmdPrompt_Ref"=w199) -> ("error out"=w196:errorcluster)  [unwired: 7 in]
        n105 = call "EnableDisableControlls.vi"("error in (no error)"=w196, "State"=w201, "Common Refs"=w207) -> ("error out"=w204:errorcluster)  [unwired: 8 in]
        n106 = call <vilib>:"Initialize.vi"("error in (no error)"=w204, "Datastrem State"=w201, "OXY_SCPI Resource In"=w203) -> ("error out"=w202:errorcluster)  [unwired: 7 in, 1 out]
        n107 = call "FGV_GraphData.vi"("Mode"=enum16{"Reset", "Add", "Get"}."Reset", "error in (no error)"=w202) -> ("error out"=w206:errorcluster)  [unwired: 8 in, 1 out]
      }
      frame "Button_StopTransfer_Pressed" {
        n108 = Unbundle By Name(w224) -> ("STR_CmdPromp"=w218:refnum<vi>, "OXY_SCPI Ref"=w219:refnum<visa-resource-name>)
        n109 = call-poly <vilib>:"Stop.vi"("error in (no error)"=w228, "Stream Group"=1, "OXY_SCPI Reseource In"=w219) -> ("error out"=w231:errorcluster, "communication_data"=w230:T10)  [unwired: 6 in, 1 out]
        n110 = call "VI_CmdPrompt.vi"("Mode"=Enum_CmdPromptActions."Add", "error in (no error)"=w231, "communication_data"=w230, "STR_CmdPrompt_Ref"=w218) -> ("error out"=w226:errorcluster)  [unwired: 7 in]
        n111 = call <vilib>:"State.vi"("error in (no error)"=w226, "Group"=1, "OXY_SCPI Reseource In"=w219) -> ("error out"=w220:errorcluster, "communication_data"=w217:T10)  [unwired: 5 in, 2 out]
        n112 = call "VI_CmdPrompt.vi"("Mode"=Enum_CmdPromptActions."Add", "error in (no error)"=w220, "communication_data"=w217, "STR_CmdPrompt_Ref"=w218) -> ("error out"=w221:errorcluster)  [unwired: 7 in]
        n113 = call "EnableDisableControlls.vi"("error in (no error)"=w221, "State"=States."Initialized", "Common Refs"=w224) -> ("error out"=w225:errorcluster)  [unwired: 8 in]
      }
      frame "Button_SetPort_Presssed" {
        n114 = Unbundle By Name(w234) -> ("STR_CmdPromp"=w235:refnum<vi>, "OXY_SCPI Ref"=w241:refnum<visa-resource-name>, "Port"=w247:refnum<vi>)
        n115 = property class="DigNum (strict)"(reference=w247, error in=w245) -> ("Value"=w246:u32)  [unwired: 2 out]
        n116 = call-poly <vilib>:"Port.vi"("Port"=w246, "Stream Group"=1, "OXY_SCPI Reseource In"=w241) -> ("error out"=w250:errorcluster, "communication_data"=w249:T10)  [unwired: 6 in, 1 out]
        n117 = call "VI_CmdPrompt.vi"("Mode"=Enum_CmdPromptActions."Add", "error in (no error)"=w250, "communication_data"=w249, "STR_CmdPrompt_Ref"=w235) -> ("error out"=w233:errorcluster)  [unwired: 7 in]
        n118 = Unbundle By Name(w234) -> ("OXY_SCPI Ref"=w242:refnum<visa-resource-name>)  [unwired: 1 out]
        n119 = call <vilib>:"State.vi"("error in (no error)"=w233, "Group"=1, "OXY_SCPI Reseource In"=w242) -> ("error out"=w239:errorcluster, "communication_data"=w238:T10, "State"=w236:T7)  [unwired: 5 in, 1 out]
        n120 = call "VI_CmdPrompt.vi"("Mode"=Enum_CmdPromptActions."Add", "error in (no error)"=w239, "communication_data"=w238, "STR_CmdPrompt_Ref"=w235) -> ("error out"=w237:errorcluster)  [unwired: 7 in]
        n121 = call "EnableDisableControlls.vi"("error in (no error)"=w237, "State"=w236, "Common Refs"=w234) -> ("error out"=w244:errorcluster)  [unwired: 8 in]
      }
      frame "Button_GetPort_Pressed" {
        n122 = Unbundle By Name(w257) -> ("STR_CmdPromp"=w255:refnum<vi>, "OXY_SCPI Ref"=w256:refnum<visa-resource-name>)
        n123 = call-poly <vilib>:"Port.vi"("error in (no error)"=w259, "Group"=1, "OXY_SCPI Reseource In"=w256) -> ("error out"=w258:errorcluster, "communication_data"=w254:T10)  [unwired: 5 in, 2 out]
        n124 = call "VI_CmdPrompt.vi"("Mode"=Enum_CmdPromptActions."Add", "error in (no error)"=w258, "communication_data"=w254, "STR_CmdPrompt_Ref"=w255) -> ("error out"=w252:errorcluster)  [unwired: 7 in]
      }
      frame "Button_GetState_Pressed" {
        n125 = Unbundle By Name(w265) -> ("STR_CmdPromp"=w262:refnum<vi>, "OXY_SCPI Ref"=w264:refnum<visa-resource-name>)
        n126 = call <vilib>:"State.vi"("error in (no error)"=w269, "Group"=1, "OXY_SCPI Reseource In"=w264) -> ("error out"=w267:errorcluster, "communication_data"=w261:T10)  [unwired: 5 in, 2 out]
        n127 = call "VI_CmdPrompt.vi"("Mode"=Enum_CmdPromptActions."Add", "error in (no error)"=w267, "communication_data"=w261, "STR_CmdPrompt_Ref"=w262) -> ("error out"=w266:errorcluster)  [unwired: 7 in]
      }
      frame "Button_Init_Pressed" {
        n128 = Unbundle By Name(w274) -> ("STR_CmdPromp"=w293:refnum<vi>, "OXY_SCPI Ref"=w301:refnum<visa-resource-name>)
        n129 = Unbundle By Name(w274) -> ("STR_ChName1"=w311:refnum<vi>, "STR_ChName2"=w312:refnum<vi>, "STR_ChName3"=w314:refnum<vi>, "STR_ChName4"=w313:refnum<vi>, "STR_ChName5"=w310:refnum<vi>, "STR_ChName6"=w309:refnum<vi>)
        n130 = Build Array(w311, w312, w314, w313, w310, w309) -> (w308:refnum<vi>[])
        n131 = for {
          tunnel: w308 -> [w343] mode=indexing
          tunnel: [w345] -> w299 mode=indexing if=w342
          n132 = property class="Str"(reference=w343) -> ("Value"=w345:string)  [unwired: 1 in, 2 out]
          n133 = String Length(string=w345) -> (length=w344:i32)
          n134 = Greater Than 0?(x=w344) -> (x > 0?=w342:bool)
        }
        n135 = call-poly <vilib>:"Items.vi"("error in (no error)"=w302, "Channels"=w299, "Stream Group"=1, "OXY_SCPI Reseource In"=w301) -> ("error out"=w306:errorcluster, "communication_data"=w307:T10, "OXY_SCPI Reseource Out"=w300:refnum<visa-resource-name>)  [unwired: 5 in]
        n136 = call "VI_CmdPrompt.vi"("Mode"=Enum_CmdPromptActions."Add", "error in (no error)"=w306, "communication_data"=w307, "STR_CmdPrompt_Ref"=w293) -> ("error out"=w303:errorcluster)  [unwired: 7 in]
        n137 = Unbundle By Name(w274) -> ("STR_ConnAddress"=w271:refnum<vi>, "Port"=w286:refnum<vi>, "OXY_SCPI Ref"=w272:refnum<visa-resource-name>, "DS Ref"=w270:refnum<visa-resource-name>)
        n138 = call-poly <vilib>:"Init.vi"("error in (no error)"=w303, "Stream Group"=1, "OXY_SCPI Reseource In"=w300) -> ("error out"=w316:errorcluster, "communication_data"=w297:T10)  [unwired: 6 in, 1 out]
        n139 = call "VI_CmdPrompt.vi"("Mode"=Enum_CmdPromptActions."Add", "error in (no error)"=w316, "communication_data"=w297, "STR_CmdPrompt_Ref"=w293) -> ("error out"=w275:errorcluster)  [unwired: 7 in]
        n140 = property class="DigNum (strict)"(reference=w286) -> ("Value"=w285:u32)  [unwired: 1 in, 2 out]
        n141 = flat-sequence {
          tunnel: w275 -> [w321]
          tunnel: [w321] -> w288
          tunnel: [w328] -> w277
          tunnel: w280 -> [w327]
          tunnel: [w326] -> w279
          tunnel: w288 -> [w323]
          tunnel: w270 -> [w322]
          frame #0 {
            n142 = Wait (ms)(milliseconds to wait=u32 100) -> ()  [unwired: 1 out]
          }
          frame #1 {
            n143 = call <vilib>:"Disconnect Datastream Port.vi"("error in (no error)"=w323, "OXY_SCPI Reseource Out"=w322) -> ("error out"=w325:errorcluster)  [unwired: 9 in]
            n144 = call <vilib>:"Clear Errors.vi"("error in (no error)"=w325) -> ("error out"=w324:errorcluster)  [unwired: 5 in, 1 out]
            n145 = call <vilib>:"Connect Datastream Port.vi"("error in (no error)"=w324, "OXY_SCPI Resource In"=w327) -> ("error out"=w326:errorcluster, "OXY_SCPI Resource Out"=w328:refnum<visa-resource-name>)  [unwired: 8 in]
          }
        }
        n146 = property on="Property Node" class="Str"(reference=w271) -> ("Value"=w281:string)  [unwired: 1 in, 2 out]
        n147 = Match Pattern(string=w281, regular expression=":") -> (before substring=w284:string, match substring=w283:string)  [unwired: 1 in, 2 out]
        n148 = Number To Decimal String(number=w285) -> (decimal integer string=w282:string)  [unwired: 1 in]
        n149 = Concatenate Strings(w284, w283, w282) -> (w280:string)
        n150 = case shown="No Error" w279 {
          selector: w279 -> [w318 _]
          tunnel: [w319 _] -> w278
          tunnel: w277 -> [w319 _]
          tunnel: [w318 _] -> w273
          frame No Error {
          }
          frame Error {
          }
        }
        n151 = Bundle By Name(cluster=w274, "DS Ref"=w278) -> (w276:T3)
        n152 = flat-sequence {
          tunnel: w293 -> [w330]
          tunnel: w272 -> [w331]
          tunnel: w273 -> [w332]
          tunnel: [w332] -> w291
          tunnel: [w331] -> w290
          tunnel: [w330] -> w289
          tunnel: [w338] -> w295
          tunnel: [w333] -> w292
          tunnel: w291 -> [w340]
          tunnel: w290 -> [w339]
          tunnel: w289 -> [w336]
          frame #0 {
            n153 = Wait (ms)(milliseconds to wait=u32 50) -> ()  [unwired: 1 out]
          }
          frame #1 {
            n154 = call <vilib>:"State.vi"("error in (no error)"=w340, "Group"=1, "OXY_SCPI Reseource In"=w339) -> ("error out"=w334:errorcluster, "communication_data"=w335:T10, "State"=w338:T7)  [unwired: 5 in, 1 out]
            n155 = call "VI_CmdPrompt.vi"("Mode"=Enum_CmdPromptActions."Add", "error in (no error)"=w334, "communication_data"=w335, "STR_CmdPrompt_Ref"=w336) -> ("error out"=w333:errorcluster)  [unwired: 7 in]
          }
        }
        n156 = Unbundle By Name(w276) -> ("DS Ref"=w294:refnum<visa-resource-name>)
        n157 = call <vilib>:"Initialize.vi"("error in (no error)"=w292, "Datastrem State"=w295, "OXY_SCPI Resource In"=w294) -> ("error out"=w296:errorcluster)  [unwired: 7 in, 1 out]
        n158 = call "EnableDisableControlls.vi"("error in (no error)"=w296, "State"=w295, "Common Refs"=w276) -> ("error out"=w298:errorcluster)  [unwired: 8 in]
      }
    }
  }
  n159 = while {
    tunnel: w5 -> [w393]
    tunnel: w3 -> [w389]
    tunnel: w2 -> [w367]
    stop <- w390 stop-if-true
    n160 = Dequeue Element(queue=w367, timeout in ms (-1)=10) -> (element=w364:T2[])  [unwired: 1 in, 3 out]
    n161 = Unbundle By Name(w389) -> ("Graph"=w370:refnum<vi>)
    n162 = Preview Queue Element(queue=w393) -> (element=w392:T4)  [unwired: 2 in, 3 out]
    n163 = Equal?(x=w392, y=Enum_MainQueueElements."CloseApp") -> (x = y?=w390:bool)
    n164 = call-by-ref "?"("Mode"=enum16{"Reset", "Add", "Get"}."Add", "Data"=w364) -> ("error out"=w365:errorcluster, "Data out"=w368:T2[])  [unwired: 10 in, 2 out]
    n165 = Index Array(array=w368) -> (element #1=w388:T2, element #2=w380:T2, element #3=w379:T2, element #4=w378:T2, element #5=w377:T2, element #6=w376:T2)  [unwired: 6 in]
    n166 = property class="XYGraph (strict)"(reference=w370, error in=w365, "Value"=w368) -> ()  [unwired: 2 out]
    n167 = Unbundle By Name(w388) -> ("DataPoints"=w351:cluster{"Time":dbl, "Value":dbl}[])
    n168 = Unbundle By Name(w380) -> ("DataPoints"=w350:cluster{"Time":dbl, "Value":dbl}[])
    n169 = Unbundle By Name(w379) -> ("DataPoints"=w349:cluster{"Time":dbl, "Value":dbl}[])
    n170 = Unbundle By Name(w376) -> ("DataPoints"=w346:cluster{"Time":dbl, "Value":dbl}[])
    n171 = Unbundle By Name(w378) -> ("DataPoints"=w348:cluster{"Time":dbl, "Value":dbl}[])
    n172 = Unbundle By Name(w377) -> ("DataPoints"=w347:cluster{"Time":dbl, "Value":dbl}[])
    n173 = Array Size(array=w349) -> (size(s)=w361:i32)
    n174 = Array Size(array=w351) -> (size(s)=w363:i32)
    n175 = Array Size(array=w348) -> (size(s)=w360:i32)
    n176 = Array Size(array=w346) -> (size(s)=w358:i32)
    n177 = Array Size(array=w350) -> (size(s)=w362:i32)
    n178 = Array Size(array=w347) -> (size(s)=w359:i32)
    n179 = Decrement(x=w361) -> (x-1=w354:i32)
    n180 = Decrement(x=w363) -> (x-1=w352:i32)
    n181 = Decrement(x=w360) -> (x-1=w355:i32)
    n182 = Decrement(x=w358) -> (x-1=w357:i32)
    n183 = Decrement(x=w362) -> (x-1=w353:i32)
    n184 = Decrement(x=w359) -> (x-1=w356:i32)
    n185 = Index Array(array=w351, index=w352) -> (element=w387:cluster{"Time":dbl, "Value":dbl})
    n186 = Index Array(array=w350, index=w353) -> (element=w385:cluster{"Time":dbl, "Value":dbl})
    n187 = Index Array(array=w349, index=w354) -> (element=w384:cluster{"Time":dbl, "Value":dbl})
    n188 = Index Array(array=w348, index=w355) -> (element=w383:cluster{"Time":dbl, "Value":dbl})
    n189 = Index Array(array=w346, index=w357) -> (element=w381:cluster{"Time":dbl, "Value":dbl})
    n190 = Index Array(array=w347, index=w356) -> (element=w382:cluster{"Time":dbl, "Value":dbl})
    n191 = Unbundle By Name(w387) -> ("Value"=→"Num_ChValue1":dbl)
    n192 = Unbundle By Name(w385) -> ("Value"=→"Num_ChValue2":dbl)
    n193 = Unbundle By Name(w384) -> ("Value"=→"Num_ChValue3":dbl)
    n194 = Unbundle By Name(w383) -> ("Value"=→"Num_ChValue4":dbl)
    n195 = Unbundle By Name(w381) -> ("Value"=→"Num_ChValue6":dbl)
    n196 = Unbundle By Name(w382) -> ("Value"=→"Num_ChValue5":dbl)
  }
  n197 = while {
    tunnel: w5 -> [w395]
    tunnel: w34 -> [w397]
    stop <- FALSE stop-if-true
    n198 = event shown="[12] \"Button_Disconnect\": Value Change" {
      selector: _ -> [_ _ _ _ _ _ _ _ _ _ _ _ _ _ _ _ _]
      dyn-events: _ -> [_ _ _ _ _ _ _ _ _ _ _ _ _ _ _ _ _]
      timeout: 100 -> [_ _ _ _ _ _ _ _ _ _ _ _ _ _ _ _ _]
      tunnel: w395 -> [w398 w404 w408 w412 w414 w418 w422 w426 w430 w435 w440 w454 w468 _ _ w484 w504]
      tunnel: w397 -> [w401 w403 w407 w411 w416 w420 w424 w428 w432 w436 w439 w453 w467 _ _ w486 w502]
      tunnel: [w400 w402 w406 w410 w415 w419 w423 w427 w431 w434 w438 w452 w466 _ _ w485 _] -> _
      event Timeout {
        n199 = event-data() -> ()  [unwired: 1 in, 3 out]
        n200 = Enqueue Element(queue=w398, element=Enum_MainQueueElements."Timeout", error in (no error)=w401) -> (error out=w400:errorcluster)  [unwired: 1 in, 2 out]
      }
      event "Button_Start": Value Change {
        n201 = event-data() -> ()  [unwired: 1 in, 3 out]
        n202 = Enqueue Element(queue=w404, element=Enum_MainQueueElements."Button_StartTransfer_Pressed", error in (no error)=w403) -> (error out=w402:errorcluster)  [unwired: 1 in, 2 out]
      }
      event "Button_Stop": Value Change {
        n203 = event-data() -> ()  [unwired: 1 in, 3 out]
        n204 = Enqueue Element(queue=w408, element=Enum_MainQueueElements."Button_StopTransfer_Pressed", error in (no error)=w407) -> (error out=w406:errorcluster)  [unwired: 1 in, 2 out]
      }
      event "Button_Connect": Value Change {
        n205 = event-data() -> ()  [unwired: 1 in, 3 out]
        n206 = Enqueue Element(queue=w412, element=Enum_MainQueueElements."Button_Connect_Pressed", error in (no error)=w411) -> (error out=w410:errorcluster)  [unwired: 1 in, 2 out]
      }
      event "Button_querryChs": Value Change {
        n207 = event-data() -> ()  [unwired: 1 in, 6 out]
        n208 = Enqueue Element(queue=w414, element=Enum_MainQueueElements."Button_QuerryChList_Pressed", error in (no error)=w416) -> (error out=w415:errorcluster)  [unwired: 1 in, 2 out]
      }
      event "Button_Set_Port": Value Change {
        n209 = event-data() -> ()  [unwired: 1 in, 6 out]
        n210 = Enqueue Element(queue=w418, element=Enum_MainQueueElements."Button_SetPort_Presssed", error in (no error)=w420) -> (error out=w419:errorcluster)  [unwired: 1 in, 2 out]
      }
      event "Button_Get_Port": Value Change {
        n211 = event-data() -> ()  [unwired: 1 in, 6 out]
        n212 = Enqueue Element(queue=w422, element=Enum_MainQueueElements."Button_GetPort_Pressed", error in (no error)=w424) -> (error out=w423:errorcluster)  [unwired: 1 in, 2 out]
      }
      event "Button_Get_State": Value Change {
        n213 = event-data() -> ()  [unwired: 1 in, 6 out]
        n214 = Enqueue Element(queue=w426, element=Enum_MainQueueElements."Button_GetState_Pressed", error in (no error)=w428) -> (error out=w427:errorcluster)  [unwired: 1 in, 2 out]
      }
      event "Button_Init": Value Change {
        n215 = event-data() -> ()  [unwired: 1 in, 6 out]
        n216 = Enqueue Element(queue=w430, element=Enum_MainQueueElements."Button_Init_Pressed", error in (no error)=w432) -> (error out=w431:errorcluster)  [unwired: 1 in, 2 out]
      }
      event "Button_Reset": Value Change {
        n217 = event-data() -> ()  [unwired: 1 in, 6 out]
        n218 = Enqueue Element(queue=w435, element=Enum_MainQueueElements."Button_Reset_Pressed", error in (no error)=w436) -> (error out=w434:errorcluster)  [unwired: 1 in, 2 out]
      }
      event "STR_HostAddress": Key Down {
        n219 = event-data() -> ("VKey"=w441:T11)  [unwired: 1 in]
        n220 = Equal?(x=w441, y=eventvkey."Enter") -> (x = y?=w443:bool)
        n221 = Equal?(x=w441, y=eventvkey."Return") -> (x = y?=w444:bool)
        n222 = Or(x=w444, y=w443) -> (x .or. y?=w442:bool)
        n223 = case shown="True" w442 {
          tunnel: w440 -> [_ w450]
          tunnel: [w447 w449] -> w438
          tunnel: w439 -> [w447 w448]
          frame False {
          }
          frame True {
            n224 = Enqueue Element(queue=w450, element=Enum_MainQueueElements."Button_Connect_Pressed", error in (no error)=w448) -> (error out=w449:errorcluster)  [unwired: 1 in, 2 out]
          }
        }
      }
      event "User Commands": Key Down {
        n225 = event-data() -> ("VKey"=w455:T11)  [unwired: 1 in]
        n226 = Equal?(x=w455, y=eventvkey."Enter") -> (x = y?=w457:bool)
        n227 = Equal?(x=w455, y=eventvkey."Return") -> (x = y?=w458:bool)
        n228 = Or(x=w458, y=w457) -> (x .or. y?=w456:bool)
        n229 = case shown="True" w456 {
          tunnel: w454 -> [_ w464]
          tunnel: [w461 w463] -> w452
          tunnel: w453 -> [w461 w462]
          frame False {
          }
          frame True {
            n230 = Enqueue Element(queue=w464, element=Enum_MainQueueElements."Button_UsrCmdSet_Pressed", error in (no error)=w462) -> (error out=w463:errorcluster)  [unwired: 1 in, 2 out]
          }
        }
      }
      event "Button_Disconnect": Value Change {
        n231 = event-data() -> ()  [unwired: 1 in, 3 out]
        n232 = Enqueue Element(queue=w468, element=Enum_MainQueueElements."Button_Disconnect_Pressed", error in (no error)=w467) -> (error out=w466:errorcluster)  [unwired: 1 in, 2 out]
      }
      event "LBox_ChList": Drag Starting? {
        n233 = event-data() -> ("CtlRef"=w476:refnum<vi>)  [unwired: 1 in]
        n234 = property on="Property Node" class="MCListbox (strict)"(reference=w476) -> ("Value"=w473:i32, "ItemNames"=w470:string[][])  [unwired: 1 in, 2 out]
        n235 = Index Array(array=w470, index (row)=w473, index (col)=0 ("disabled index (col)")) -> (element=w471:string)
        n236 = To Variant(anything=w471) -> (Variant=w479:variant)
        n237 = Bundle("DragChannel", "Variant"=w479) -> (w477:cluster{string, "Variant":variant})  [unwired: 1 in]
        n238 = Build Array(w477) -> (w474:cluster{string, "Variant":variant}[])
        n239 = event-data("Data"=w474, "Drag Mode"=enum32{"copy or move", "copy only", "move only"}."copy only") -> ()  [unwired: 1 in, 1 out]
      }
      event "STR_ChName1", "STR_ChName2", "STR_ChName3", "STR_ChName4", "STR_ChName5", "STR_ChName6": Drag Enter {
        n240 = event-data() -> ("Available Data Names"=w482:string[])  [unwired: 1 in, 1 out]
        n241 = Search 1D Array(1D array=w482, element="DragChannel") -> (index of element=w483:i32)  [unwired: 1 in]
        n242 = Greater Or Equal To 0?(x=w483) -> (x >= 0?=w480:bool)
        n243 = event-data("Accepted?"=w480) -> ()  [unwired: 1 in, 1 out]
      }
      event "STR_ChName1", "STR_ChName2", "STR_ChName3", "STR_ChName4", "STR_ChName5", "STR_ChName6": Drop {
        w494 = "DragChannel"
        n244 = event-data() -> ("CtlRef"=w489:refnum<vi>, "Available Data Names"=w493:string[])  [unwired: 1 in]
        n245 = Search 1D Array(1D array=w493, element=w494) -> (index of element=w495:i32)  [unwired: 1 in]
        n246 = case shown="Default" w495 {
          tunnel: w494 -> [_ w501]
          tunnel: [FALSE TRUE] -> w492
          tunnel: [" " w498] -> w490
          frame Default {
          }
          frame 0.. {
            n247 = Get Drag Drop Data(8:"", 9:w501) -> (3:w498:string)  [unwired: 1 in, 1 out]
          }
        }
        n248 = call "FGV_DrapAndDrop_Data.vi"("Modes"=TD_Case_SimpleFGVModes."Set", "error in (no error)"=w486, "Target String Element Ref"=w489, "Channel Name"=w490) -> ("error out"=w487:errorcluster)  [unwired: 5 in, 2 out]
        n249 = Enqueue Element(queue=w484, element=Enum_MainQueueElements."NewDragAndDrop", error in (no error)=w487) -> (error out=w485:errorcluster)  [unwired: 1 in, 2 out]
        n250 = event-data("Accepted?"=w492) -> ()  [unwired: 1 in, 1 out]
      }
      event Application Instance Close {
        n251 = event-data() -> ()  [unwired: 1 in, 4 out]
        n252 = Enqueue Element(queue=w504, element=Enum_MainQueueElements."CloseApp", error in (no error)=w502) -> ()  [unwired: 1 in, 3 out]
      }
    }
  }
  "Recorder" <- T2[] [] ("Data out")
